vi "Write Crypto Library Path.vi"(8 "error in (no error)":errorcluster, 10 "Crypto Library Path":path=path "C:/Program Files (x86)/National Instruments/Shared/nissl/NIlibeay32.dll", 11 "SSL-Lib in":refnum<class "SSL-Lib.lvclass">) -> (0 "error out":errorcluster, 3 "SSL-Lib out":refnum<class "SSL-Lib.lvclass">)   [LabVIEW 2013, in "OpenSSL Socket.lvlib" / "SSL-Lib.lvclass"]
uses:
  SSL-Lib.lvclass
  SSL-Lib.lvclass/SSL-Lib.ctl
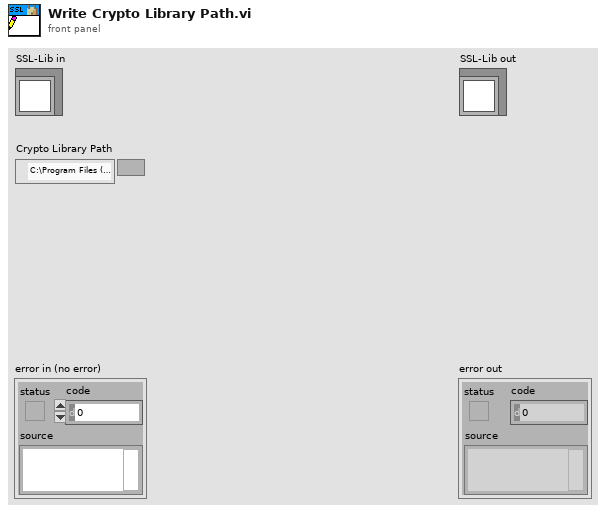
[diagram p1: front panel]
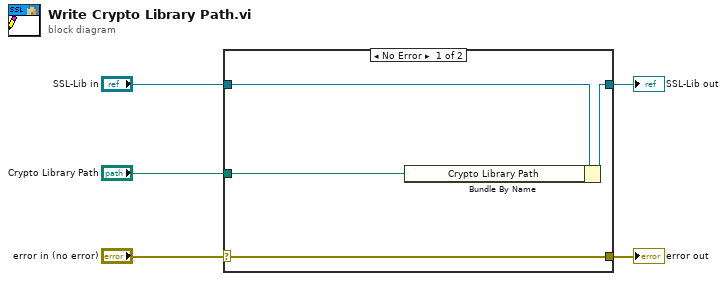
[diagram p0: block diagram]
diagram:
  n1 = case shown="No Error" "error in (no error)" {
    selector: "error in (no error)" -> [w9 w10]
    tunnel: [w9 w10] -> w4
    tunnel: [w7 w11] -> w2
    tunnel: "SSL-Lib in" -> [w8 w11]
    tunnel: "Crypto Library Path" -> [w6 _]
    frame No Error {
      n2 = Bundle By Name(cluster=w8, "Crypto Library Path"=w6) -> (w7:refnum<class "SSL-Lib.lvclass">)
    }
    frame Error {
    }
  }
  "error out" <- w4
  "SSL-Lib out" <- w2
